vi "Get UTC Offset__ogtk.vi"() -> (1 "UTC Offset String":string, 2 "UTC Offset (seconds)":i32)   [LabVIEW 2023, in "openg_variant.lvlib"]
doc: "EasyXML Toolkit for LabVIEW version 3.0.0.170\nCopyright (c) 2016, JKI. All Rights Reserved."
uses:
  openg_variant.lvlib
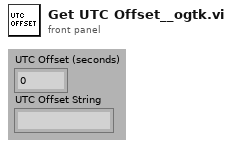
[diagram p1: front panel]
types:
  T1 = cluster{"second":i32, "minute":i32, "hour":i32, "day of month":i32, "month":i32, "year":i32, "day of week":i32, "day of year":i32, "is DST":i32}
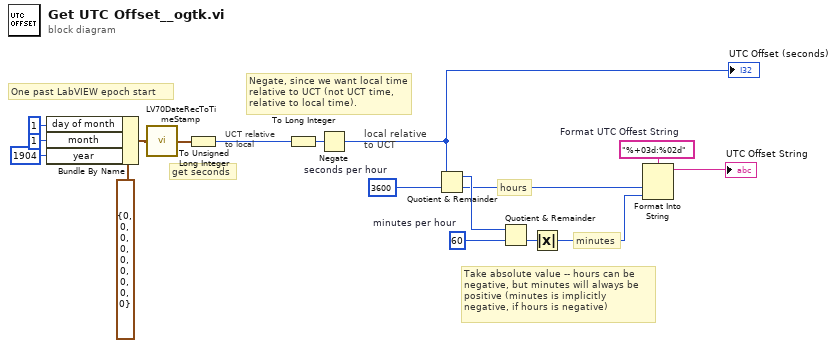
[diagram p0: block diagram]
diagram:
  w13 = 60  # minutes per hour
  w15 = 3600  # seconds per hour
  w16 = "%+03d:%02d"  # Format UTC Offest String
  # "One past LabVIEW epoch start"
  # "local relative to UCT"
  # "UCT relative to local"
  # "get seconds"
  # "Negate, since we want local time relative to UCT (not UCT time, relative to local time)."
  # "Take absolute value -- hours can be negative, but minutes will always be positive (minutes is implicitly negative, if hours is negative)"
  # "minutes"
  # "hours"
  n1 = Bundle By Name(cluster=T1 {"second"=0, "minute"=0, "hour"=0, "day of month"=0, "month"=0, "year"=0, "day of week"=0, "day of year"=0, "is DST"=0} ("date time rec"), "day of month"=1, "month"=1, "year"=1904) -> (w2:T1)
  n2 = call <vilib>:"LV70DateRecToTimeStamp.vi"("date time rec"=w2) -> ("Time Stamp"=w10:timestamp)
  n3 = To Unsigned Long Integer(number=w10) -> (unsigned 32bit integer=w17:u32)
  n4 = To Long Integer(number=w17) -> (32bit integer=w8:i32)
  n5 = Negate(x=w8) -> (-x=w7:i32)
  "UTC Offset (seconds)" <- w7
  n6 = Quotient & Remainder(x=w7, y=w15) -> (x-y*floor(x/y)=w14:i32, floor(x/y)=w11:i32)
  n7 = Quotient & Remainder(x=w14, y=w13) -> (floor(x/y)=w9:i32)  [unwired: 1 out]
  n8 = Absolute Value(x=w9) -> (abs(x)=w12:i32)
  n9 = Format Into String(format string=w16, w11, w12) -> (resulting string=→"UTC Offset String":string)  [unwired: 2 in, 1 out]
